vi "CreateShapePoly.vi"   [LabVIEW 2017]
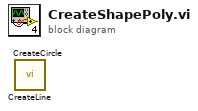
[diagram p0: block diagram]
diagram:
  n1 = call "CreateLine.vi"() -> ()  [unwired: 12 in]
  n2 = call "CreateCircle.vi"() -> ()  [unwired: 12 in]
